vi "PictureScaleFactor.vi"() -> ()   [LabVIEW 2011]
panel:
  in  "Scale Factor":dbl
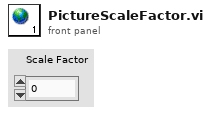
[diagram p1: front panel]
diagram:
